vi "GetActiveFieldName.vi"(1 "protobuf index":i32) -> (0 "oneof field name":string)   [LabVIEW 2019, in "grpc-xnet_client.lvlib" / "nixnet_grpc_LinDiagnosticScheduleChangeRequest_schedule_enum.lvclass"]
uses:
  nixnet_grpc_LinDiagnosticScheduleChangeRequest_schedule_enum.lvclass
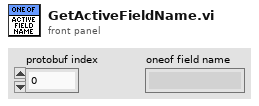
[diagram p1: front panel]
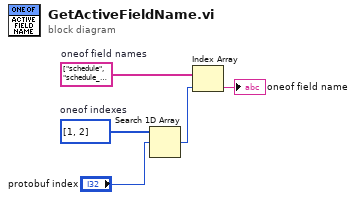
[diagram p0: block diagram]
diagram:
  w5 = string[] ["schedule", "schedule_raw"]  # oneof field names
  w4 = i32[] [1, 2]  # oneof indexes
  n1 = Search 1D Array(1D array=w4, element="protobuf index") -> (index of element=w2:i32)  [unwired: 1 in]
  n2 = Index Array(array=w5, index=w2) -> (element=→"oneof field name":string)
